vi "Base64toSGL.vi"(8 "error in (no error)":errorcluster, 10 "Base64 String":string) -> (0 "error out":errorcluster, 2 "SGL Array":sgl[](array[numeric])=[0.0, 0.0, 0.0, 0.0, 0.0, 0.0, 33.0])   [LabVIEW 2011]
doc: "This VI converts a Base 64 string to its string equivalent. Base64 strings are commonly used in Internet protocols such as HTTP, SMTP, etc."
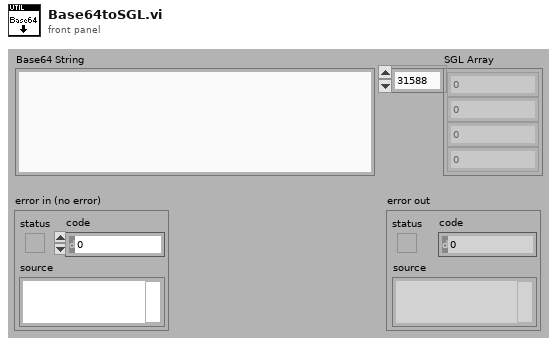
[diagram p1: front panel]
types:
  T1 = enum16{"big-endian, network order", "native, host order", "little-endian"}
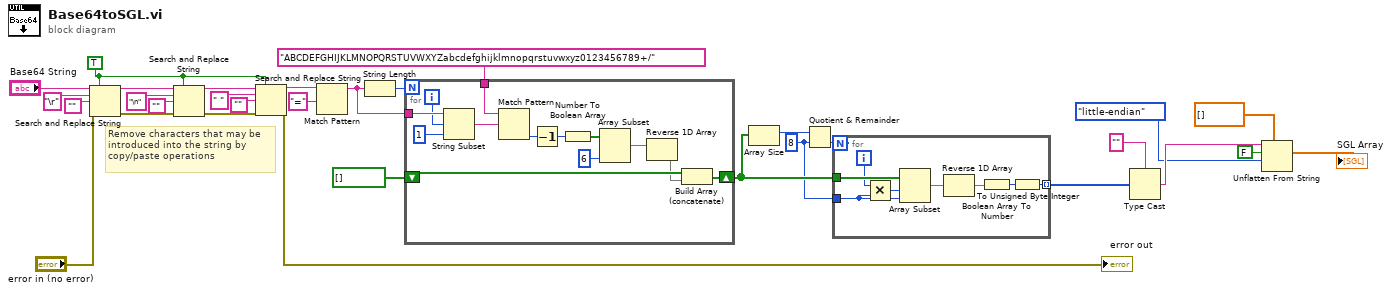
[diagram p0: block diagram]
diagram:
  w9 = TRUE ("replace all? (F)")
  w7 = 8 ("y")
  # "Remove characters that may be\nintroduced into the string by\ncopy/paste operations"
  n1 = Search and Replace String(replace all?=w9, input string="Base64 String", search string="\r" ("replace string (\"\")"), replace string="", error in="error in (no error)") -> (result string=w19:string, error out=w17:errorcluster)  [unwired: 5 out]
  n2 = Search and Replace String(replace all?=w9, input string=w19, search string="\n" ("replace string (\"\")"), replace string="", error in=w17) -> (result string=w13:string, error out=w12:errorcluster)  [unwired: 5 out]
  n3 = Search and Replace String(replace all?=w9, input string=w13, search string=" " ("replace string (\"\")"), replace string="", error in=w12) -> (result string=w10:string, error out=→"error out":errorcluster)  [unwired: 5 out]
  n4 = Match Pattern(string=w10, regular expression="=") -> (before substring=w28:string)  [unwired: 4 out]
  n5 = String Length(string=w28) -> (length=w31:i32)
  n6 = for {
    N: w31 -> [_]
    tunnel: w28 -> [w44]
    tunnel: "ABCDEFGHIJKLMNOPQRSTUVWXYZabcdefghijklmnopqrstuvwxyz0123456789+/" -> [w41]
    shift-right: [w34] -> w24
    shift-left: bool[] [] -> [w33]
    i -> [w42]
    n7 = String Subset(string=w44, offset (0)=w42, length (rest)=1 ("length (rest)")) -> (substring=w40:string)
    n8 = Match Pattern(string=w41, regular expression=w40) -> (offset past match=w39:i32)  [unwired: 1 in, 3 out]
    n9 = Decrement(x=w39) -> (x-1=w38:i32)
    n10 = Number To Boolean Array(number=w38) -> (Boolean array=w37:bool[])
    n11 = Array Subset(array=w37, length=6) -> (w35:bool[])  [unwired: 1 in]
    n12 = Reverse 1D Array(array=w35) -> (reversed array=w32:bool[])
    n13 = Build Array (concatenate)(w33, w32) -> (w34:bool[])
  }
  n14 = Array Size(array=w24) -> (size(s)=w26:i32)
  n15 = Quotient & Remainder(x=w26, y=w7) -> (floor(x/y)=w25:i32)  [unwired: 1 out]
  n16 = for {
    N: w25 -> [_]
    tunnel: w24 -> [w52]
    tunnel: w7 -> [w51]
    tunnel: [w47] -> w8 mode=indexing
    i -> [w50]
    n17 = Multiply(x=w50, y=w51) -> (x*y=w45:i32)
    n18 = Array Subset(array=w52, index=w45, length=w51) -> (w49:bool[])
    n19 = Reverse 1D Array(array=w49) -> (reversed array=w46:bool[])
    n20 = Boolean Array To Number(Boolean array=w46) -> (number=w48:u32)
    n21 = To Unsigned Byte Integer(number=w48) -> (unsigned 8bit integer=w47:u8)
  }
  n22 = Type Cast(type="", x=w8) -> (*(type *) &x=w6:string)
  n23 = Unflatten From String(type=sgl[] [], binary string=w6, data includes array or string size? (T)=FALSE, byte order (0:big-endian, network order)=T1."little-endian") -> (value=→"SGL Array":sgl[])  [unwired: 1 in, 2 out]
